vi "uintStringToUint.vi"(8 "Error in (no error)":errorcluster, 9 "String format (decimal)":T1=10 items=["Binary"=2, "Octal"=8, "Decimal"=10, "Hexadecimal"=16, "Hexatrigesimal"=36, "ASCII"=64], 10 "String in":string) -> (0 "Error out":errorcluster, 3 "Uint out":refnum<class "UintClass.lvclass">)   [LabVIEW 2011, in "UintClass.lvclass"]
uses:
  UintClass.lvclass
  enumBase.ctl
  UintClass.lvclass/UintClass.ctl
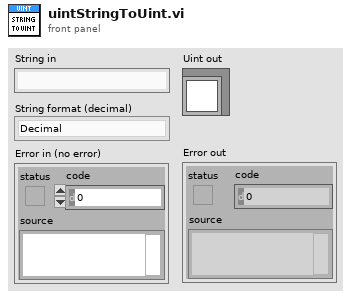
[diagram p1: front panel]
types:
  T1 = typedef "UintClass.lvclass/enumBase.ctl" = u16
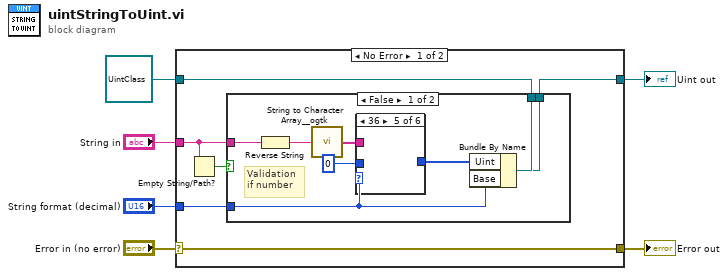
[diagram p0: block diagram]
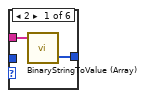
[diagram p2: hidden frame]
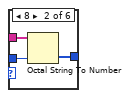
[diagram p3: hidden frame]
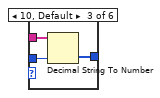
[diagram p4: hidden frame]
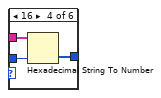
[diagram p5: hidden frame]
diagram:
  n1 = case shown="No Error" "Error in (no error)" {
    selector: "Error in (no error)" -> [w12 w33]
    tunnel: [w12 w33] -> w2
    tunnel: [w10 w34] -> w6
    tunnel: refnum<class "UintClass.lvclass"> refnum ("UintClass in") -> [w11 w34]
    tunnel: "String in" -> [w8 _]
    tunnel: "String format (decimal)" -> [w9 _]
    frame No Error {
      n2 = Empty String/Path?(string/path=w8) -> (empty?=w7:bool)
      n3 = case shown="False" w7 {
        tunnel: w11 -> [w20 w32]
        tunnel: [w19 w32] -> w10
        tunnel: w9 -> [w18 _]
        tunnel: w8 -> [w14 _]
        frame False {
          # "Validation \nif number"
          n4 = Reverse String(1:w14) -> (0:w13:string)
          n5 = call <userlib>:"String to Character Array__ogtk.vi"("Input String"=w13) -> ("Character Array"=w17:string[])
          n6 = case shown="36" w18 {
            tunnel: w17 -> [w22 w25 w28 w31 _ _]
            tunnel: u8 0 ("default (0 I32)") -> [_ w24 w27 w30 _ _]
            tunnel: [w21 w23 w26 w29 _ _] -> w15
            frame 2 {
              n7 = call "BinaryStringToValue (Array).vi"("Array string"=w22) -> ("Array value"=w21:u8[])
            }
            frame 8 {
              n8 = Octal String To Number(2:w24, 4:w25) -> (0:w23:u8[])  [unwired: 1 in, 1 out]
            }
            frame 10, Default {
              n9 = Decimal String To Number(string=w28, default (0L)=w27) -> (number=w26:u8[])  [unwired: 1 in, 1 out]
            }
            frame 16 {
              n10 = Hexadecimal String To Number(string=w31, default (0uL)=w30) -> (number=w29:u8[])  [unwired: 1 in, 1 out]
            }
            frame 36 {
            }
            frame 64 {
            }
          }
          n11 = Bundle By Name(cluster=w20, "Uint"=w15, "Base"=w18) -> (w19:refnum<class "UintClass.lvclass">)
        }
        frame True {
        }
      }
    }
    frame Error {
    }
  }
  "Uint out" <- w6
  "Error out" <- w2
